vi "Square with Sign.vi"(11 "X":dbl) -> (3 "X^2":dbl)   [LabVIEW 2015]
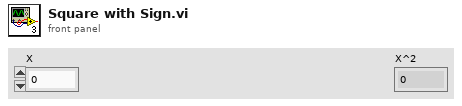
[diagram p1: front panel]
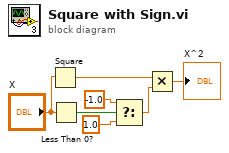
[diagram p0: block diagram]
diagram:
  n1 = Square(x="X") -> (x^2=w5:dbl)
  n2 = Less Than 0?(x="X") -> (x < 0?=w2:bool)
  n3 = Select(t=-1.0, s=w2, f=1.0) -> (s? t:f=w4:dbl)
  n4 = Multiply(x=w5, y=w4) -> (x*y=→"X^2":dbl)
